vi "Variant to Data-Imaging protocol queue.vi"(8 "error in (no error)":errorcluster, 9 "Message Data":variant) -> (0 "error out":errorcluster, 2 "Next state queue data":T1)   [LabVIEW 2017]
uses:
  Typedefs/Next state queue data.ctl
  Typedefs/Start-Stop Enum.ctl
  Typedefs/Top level VI states.ctl
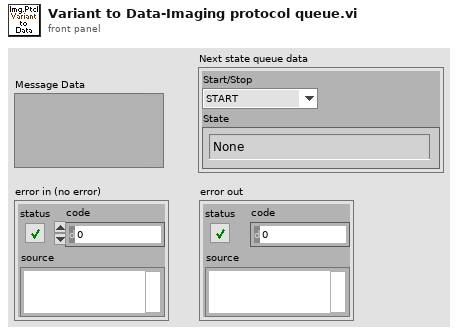
[diagram p1: front panel]
types:
  T1 = typedef "Next state queue data.ctl" = cluster{"Start/Stop":T2, "State":T3}
  T2 = typedef "Start-Stop Enum.ctl" = enum16{"START", "STOP"}
  T3 = typedef "Top level VI states.ctl" = enum16{"None", "Initialise UI", "<STACK PROTOCOL STATES>", "AOL Zstack-START", "AOL Zstack-STOP", "Motor Zstack-START", "Motor Zstack-STOP", "<ACQUISITION PROTOCOL STATES> ", "Functional Acquisition-START", "Functional Acquisition-STOP", "Single Plane Acquisition-START", "Single Plane Acquisition-STOP", "Volume Acquisition-START", "Volume Acquisition-STOP", "<LIVE IMAGING PROTOCOL STATES>", "Live Imaging-START", "Live Imaging-STOP", "Live Plane Imaging-START", "Live Plane Imaging-STOP", "Live Volume Imaging-START", "Live Volume Imaging-STOP", "<MOVEMENT CORRECTION PROTOCOL STATES>", "Background MovCor-START", "Background MovCor-STOP", "EXIT"}
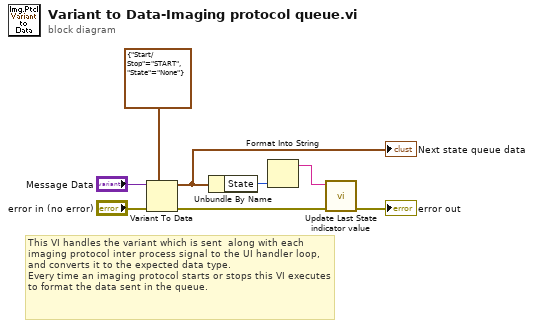
[diagram p0: block diagram]
diagram:
  # "This VI handles the variant which is sent  along with each imaging protocol inter process signal to the UI handler loop, and converts it to the expected data type.\nEvery time an imaging protocol starts or stops this VI executes to format the data sent in the queue."
  n1 = Variant To Data(error in="error in (no error)", type=T1 {"Start/Stop"=enum."START", "State"=enum."None"}, Variant="Message Data") -> (data=w3:T1, error out=w5:errorcluster)
  "Next state queue data" <- w3
  n2 = Unbundle By Name(w3) -> ("State"=w2:T3)
  n3 = Format Into String(w2) -> (resulting string=w1:string)  [unwired: 3 in, 1 out]
  n4 = call "Update Last State indicator value.vi"("error in (no error)"=w5, "Value"=w1) -> ("error out"=→"error out":errorcluster)  [unwired: 9 in]
